vi "Main.vi"() -> ()   [LabVIEW 2017]
uses:
  State/state_R.ctl
  <vilib>/daq.io/daq.io LabVIEW API/_typedefs/daqio-Credentials.ctl
  <vilib>/myRIO/Instrument Drivers/Onboard IO/DIO/typedefs/DIO Reference.ctl
  <vilib>/myRIO/Common/Instrument Driver Framework/Utilities/typedefs/myRIO Generic Hardware Reference.ctl
  <vilib>/myRIO/Common/Instrument Driver Framework/Utilities/typedefs/Hardware Version Enum.ctl
  <vilib>/myRIO/Common/Instrument Driver Framework/Utilities/typedefs/myRIO v1.0 Reference.ctl
  <vilib>/myRIO/Common/Instrument Driver Framework/Utilities/typedefs/Generic FPGA Reference.ctl
  <vilib>/myRIO/Common/Instrument Driver Framework/myRIO v1.0/DIO/typedefs/DIO Channels List.ctl
  <vilib>/myRIO/Common/Instrument Driver Framework/myRIO v1.0/DIO/typedefs/DIO Channels Enum.ctl
  <vilib>/userdefined/High Color/nirio_resource_hc.ctl
  <vilib>/myRIO/Common/Instrument Driver Framework/myRIO v1.0/DIO/vis/myRIO v1.1 Open DIO.vi
  <vilib>/myRIO/Common/Instrument Driver Framework/Utilities/vis/Validate Channels.vi
  <vilib>/myRIO/Common/Instrument Driver Framework/myRIO v1.0/DIO/vis/myRIO v1.0 Reserve DIO.vi
  <vilib>/myRIO/Common/Instrument Driver Framework/myRIO v1.0/DIO/vis/myRIO v1.0 Close DIO.vi
  <vilib>/myRIO/Common/Instrument Driver Framework/myRIO v1.0/Resource Manager/vis/myRIO v1.0 Reserve Channel List.vi
  <vilib>/myRIO/Common/Instrument Driver Framework/myRIO v1.0/DIO/vis/myRIO v1.0 Build MUX Configuration DIO.vi
  <vilib>/myRIO/Common/Instrument Driver Framework/myRIO v1.0/DIO/vis/myRIO v1.0 Unreserve DIO.vi
  <vilib>/myRIO/Common/Instrument Driver Framework/myRIO v1.0/Resource Manager/vis/myRIO v1.0 Reserve Channel.vi
  <vilib>/myRIO/Common/Instrument Driver Framework/myRIO v1.0/Resource Manager/vis/myRIO v1.0 Unreserve Channel.vi
  <vilib>/myRIO/Common/Instrument Driver Framework/myRIO v1.0/Resource Manager/vis/myRIO v1.0 Create Configuration List.vi
  <vilib>/myRIO/Common/Instrument Driver Framework/myRIO v1.0/Resource Manager/vis/myRIO v1.0 Unreserve Channel List.vi
  <vilib>/myRIO/Common/Instrument Driver Framework/myRIO v1.0/Resource Manager/vis/myRIO v1.0 Build Mutex Name.vi
  <vilib>/Utility/VariantDataType/GetNumericInfo.vi
  <vilib>/Utility/error.llb/Error Cluster From Error Code.vi
  <vilib>/myRIO/Common/Instrument Driver Framework/myRIO v1.0/myRIO v1.1 Open.vi
  <vilib>/myRIO/Common/Instrument Driver Framework/Utilities/vis/IO Manager.vi
  <vilib>/myRIO/Common/Instrument Driver Framework/Utilities/vis/Configuration Manager.vi
  <vilib>/myRIO/Common/Instrument Driver Framework/myRIO v1.0/Resource Manager/vis/myRIO v1.0 Configure IO.vi
  <vilib>/myRIO/Common/Instrument Driver Framework/myRIO v1.0/myRIO v1.0 Close.vi
  Function/Global_pH.vi
  <vilib>/daq.io/daq.io LabVIEW API/_subs/daqio_Write_Single.vi
  <vilib>/myRIO/Common/Instrument Driver Framework/myRIO v1.0/DIO/vis/myRIO v1.0 Read DIO.vi
  <vilib>/myRIO/Common/Instrument Driver Framework/myRIO v1.0/DIO/vis/myRIO v1.0 Shutdown DIO.vi
  <vilib>/myRIO/Common/Instrument Driver Framework/myRIO v1.0/DIO/vis/myRIO v1.0 Write DIO.vi
  <vilib>/myRIO/Instrument Drivers/Onboard IO/DIO/vis/myRIO DIO Open.xnode
  <vilib>/myRIO/Instrument Drivers/Onboard IO/DIO/DIO.lvlib
  <vilib>/daq.io/daq.io LabVIEW API/daqio minimal.lvlib
panel:
  in  "分割面板":enum32{"控制面板"}(tab)
  out "pH 感測器狀態異常燈號":bool
  out "pH 感測器壽命":dbl
  out "溫度(°C)":dbl
  out "溫度過高":bool
  out "溫度過低":bool
  out "溶氧飽和度過高":bool
  out "溶氧飽和度過低":bool
  in  "TEM 上限":dbl
  in  "TEM 下限":dbl
  in  "DO 上限(%)":dbl
  in  "DO 下限(%)":dbl
  out "Work":bool
  out "FREE":bool
  out "Dangerous_Work":bool
  in  "登陸設定":T1
  out "過酸":bool
  out "過鹼":bool
  in  "pH 下限":dbl
  in  "pH 上限":dbl
  out "小時":i32
  out "分":i32
  in  "量測時間設定(min)_3":i32
  in  "量測時間設定(24hr)_3":i32
  in  "量測時間設定(min)_2":i32
  in  "量測時間設定(24hr)_2":i32
  in  "量測時間設定(min)_1":i32
  in  "量測時間設定(24hr)_1":i32
  in  "控制模式":enum16{"自動", "手動"}(ring)
  in  "狀態暫停":bool
  out "LS5":bool
  out "LS4":bool
  out "LS3":bool
  out "LS2":bool
  out "LS1":bool
  in  "開始":bool
  in  "晾乾 秒數設定 (s)":dbl
  out "目前狀態":T2
  in  "pH 秒數設定(s)":dbl
  in  "噴水 秒數設定 (s)":dbl
  in  "程式終止":bool
  in  "停止動作":bool
  in  "水平-伸":bool
  in  "水平-縮":bool
  in  "垂直-降":bool
  in  "垂直-升":bool
  out "pH值":dbl
  out "量測計數(s)":dbl
  out "噴水計數(s)":dbl
  out "晾乾計數":dbl
  out "DO值(%)":dbl
  # "Automatic measurement system based on IoT"
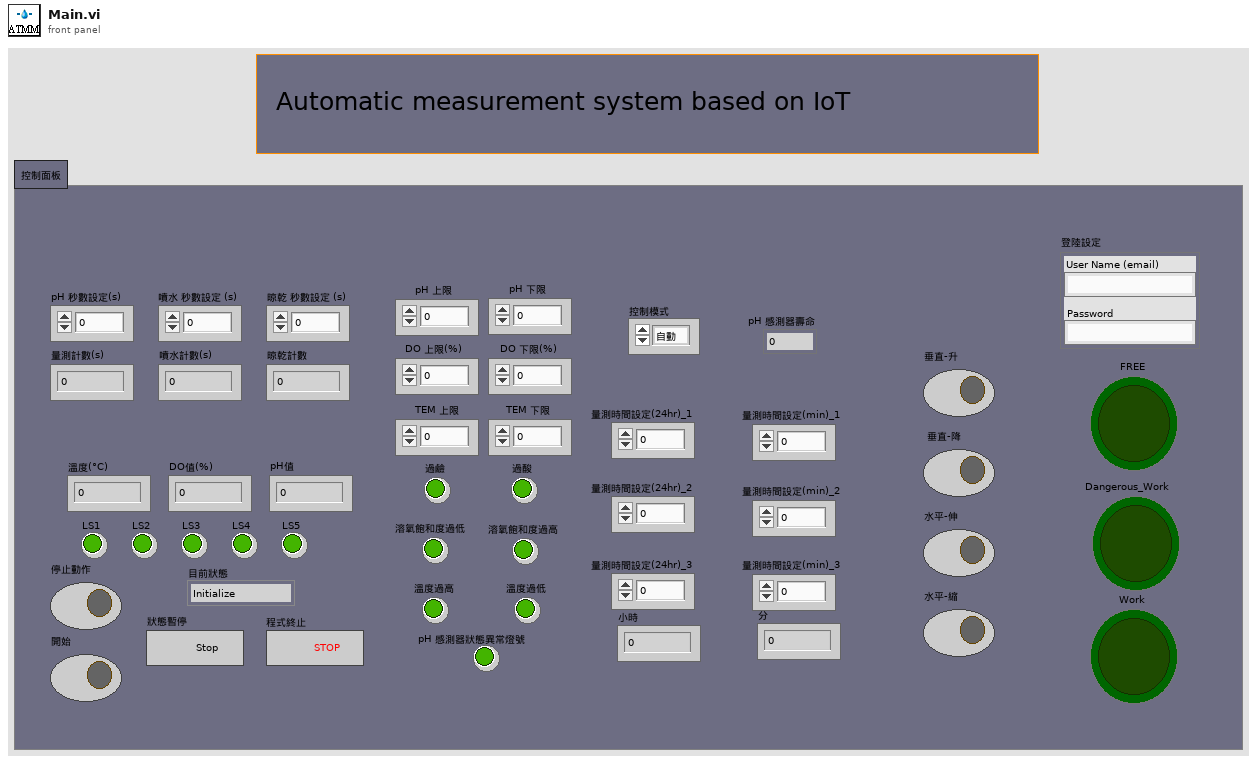
[diagram p1: front panel]
types:
  T1 = typedef "daqio minimal.lvlib/daqio-Credentials.ctl" = cluster{"User Name (email)":string, "Password":string}
  T2 = typedef "state_R.ctl" = enum16{"Initialize", "State 1", "State 2", "State 3", "State 4", "State 5", "State 6", "State 7", "State 8", "State 9", "UP", "DOWN", "EXTEND", "BACK", "Reset", "Process", "PAUSE", "Report", "Halt", "Shutdown"}
  T3 = typedef "daqio minimal.lvlib/daqio-Type.ctl" = cluster{"daq.io ref":T4, "daq.io API Base":string, "Device Key":string, "Account ID":string, "online":bool, "SSL":bool, "buffer":bool}
  T4 = typedef "LabVIEWHTTPClient.lvlib/ClientHandle.ctl" = refnum<k1>
  T5 = typedef "DIO.lvlib/DIO Reference.ctl" = cluster{"myRIO Reference":T6, "DIO Channels List":T10}
  T6 = typedef "myRIO Generic Hardware Reference.ctl" = cluster{"myRIO Model":T7, "myRIO Hardware Reference":T8}
  T7 = typedef "Hardware Version Enum.ctl" = enum16{"Unknown", "myRIO-1900", "myRIO-1950", "roboRIO", "NI ELVIS RIO CM"}
  T8 = typedef "myRIO v1.0 Reference.ctl" = cluster{"Generic FPGA Reference":T9, "Allow multiple opens":bool}
  T9 = typedef "Generic FPGA Reference.ctl" = refnum<k20>
  T10 = typedef "DIO Channels List.ctl" = T11[]
  T11 = typedef "DIO Channels Enum.ctl" = enum16{"Not Connected", "C/DIO0", "C/DIO1", "C/DIO2", "C/DIO3", "C/DIO4", "C/DIO5", "C/DIO6", "C/DIO7", "A/DIO0", "A/DIO1", "A/DIO2", "A/DIO3", "A/DIO4", "A/DIO5", "A/DIO6", "A/DIO7", "A/DIO8", "A/DIO9", "A/DIO10", "A/DIO11", "A/DIO12", "A/DIO13", "A/DIO14", "A/DIO15", "B/DIO0", "B/DIO1", "B/DIO2", "B/DIO3", "B/DIO4", "B/DIO5", "B/DIO6", "B/DIO7", "B/DIO8", "B/DIO9", "B/DIO10", "B/DIO11", "B/DIO12", "B/DIO13", "B/DIO14", "B/DIO15", "LED0", "LED1", "LED2", "LED3", "Button0", "DIO/DIO0", "DIO/DIO1", "DIO/DIO2", "DIO/DIO3", "DIO/DIO4", "DIO/DIO5", "DIO/DIO6", "DIO/DIO7", "DIO/DIO8", "DIO/DIO9", "SPI/CS0", "SPI/CS1", "SPI/CS2", "SPI/CS3", "LED RADIO (Green)", "LED RADIO (Red)", "LED COMM (Green)", "LED COMM (Red)", "LED MODE (Green)", "LED MODE (Red)"}
  T12 = typedef "LVDateTimeRec.ctl" = cluster{"fractional second":dbl, "second":i32, "minute":i32, "hour":i32, "day of month":i32, "month":i32, "year":i32, "day of week":i32, "day of year":i32, "DST":i32}
  T13 = typedef "state_D.ctl" = enum16{"Halt", "Start", "LS1", "LS2", "LS3", "LS4", "LS5", "UP", "DOWN", "EXTEND", "BACK", "Stop", "Pause"}
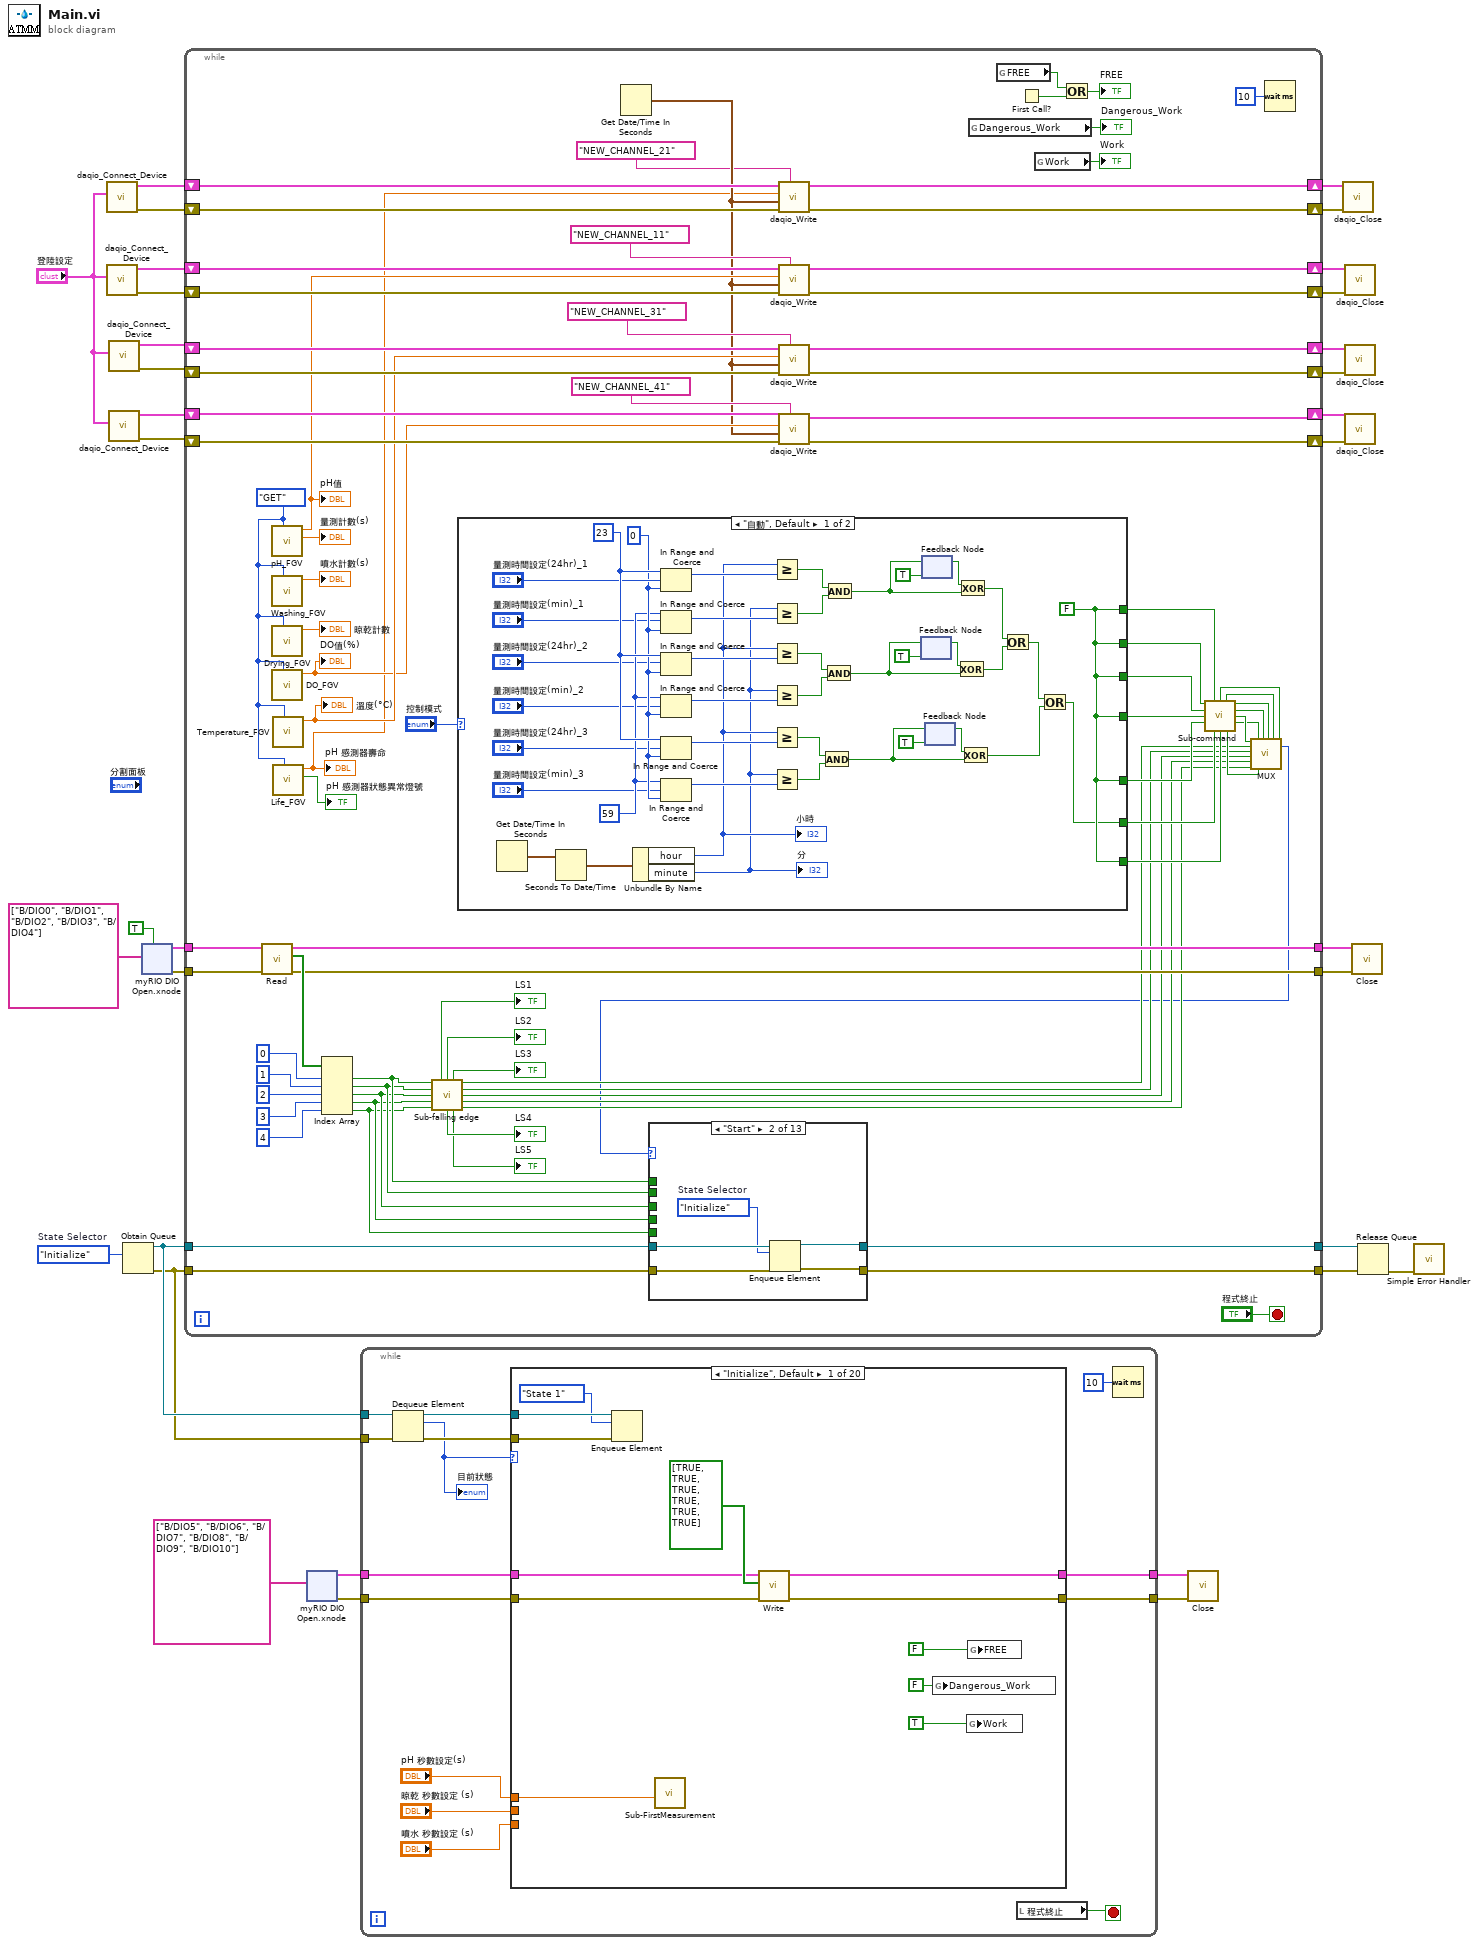
[diagram p0: block diagram]
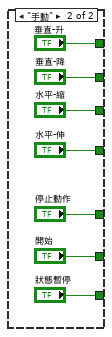
[diagram p2: hidden frame]
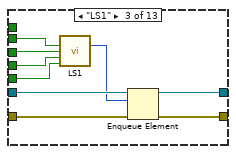
[diagram p4: hidden frame]
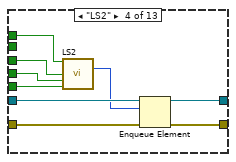
[diagram p5: hidden frame]
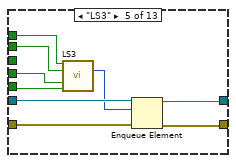
[diagram p6: hidden frame]
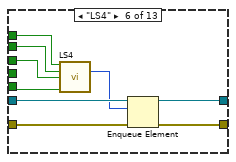
[diagram p7: hidden frame]
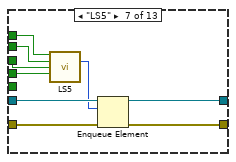
[diagram p8: hidden frame]
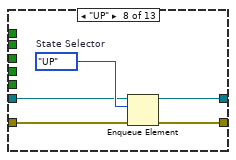
[diagram p9: hidden frame]
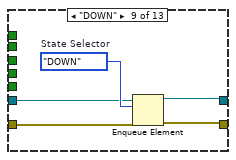
[diagram p10: hidden frame]
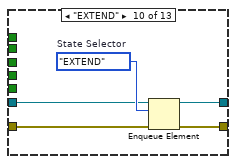
[diagram p11: hidden frame]
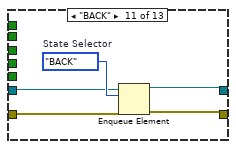
[diagram p12: hidden frame]
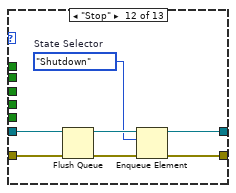
[diagram p13: hidden frame]
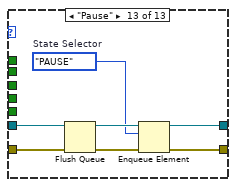
[diagram p14: hidden frame]
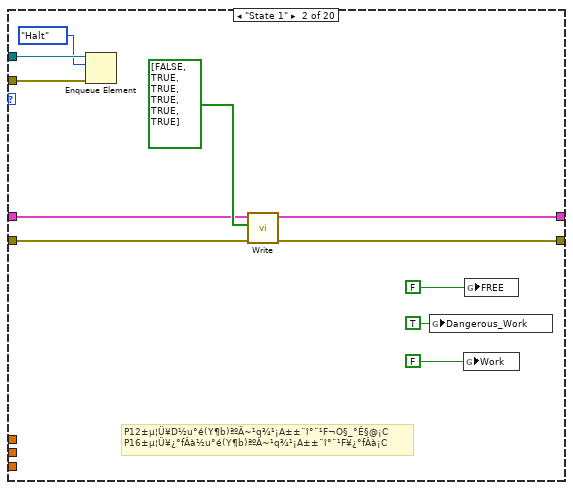
[diagram p15: hidden frame]
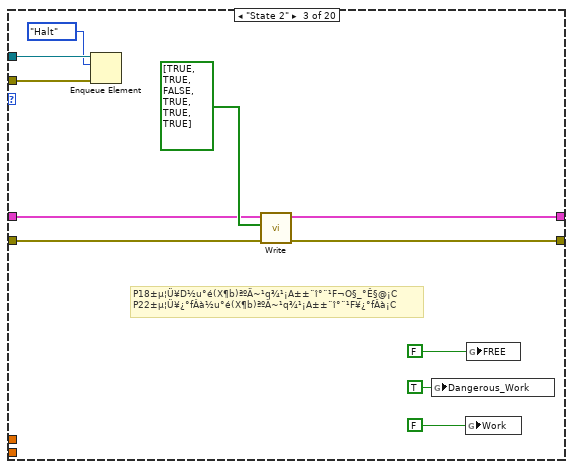
[diagram p16: hidden frame]
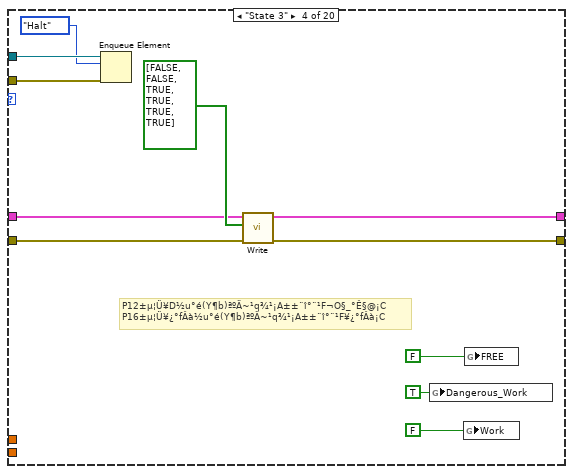
[diagram p17: hidden frame]
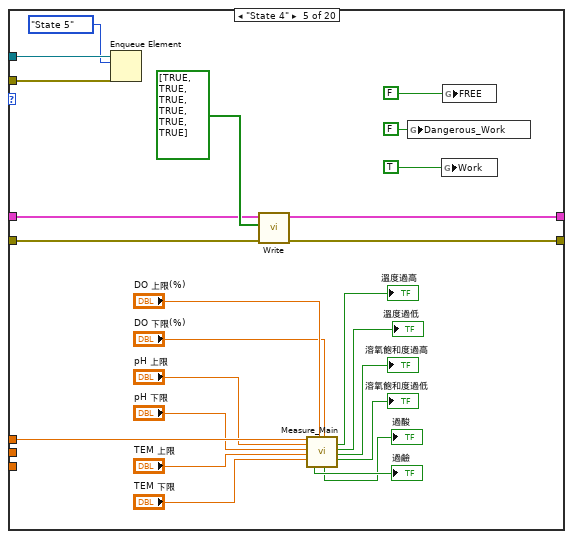
[diagram p18: hidden frame]
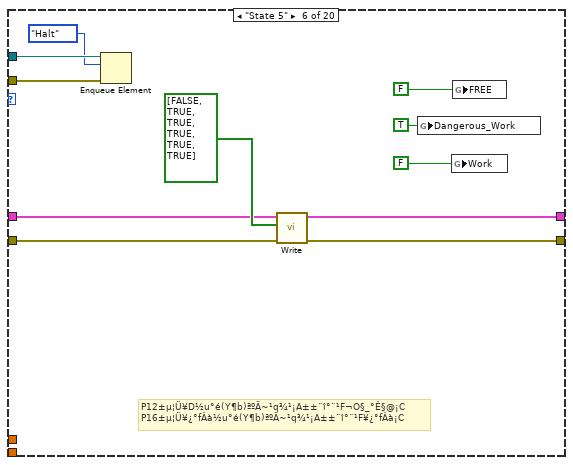
[diagram p19: hidden frame]
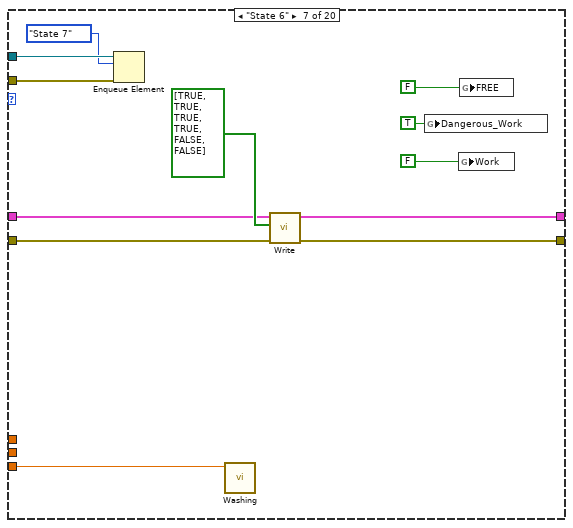
[diagram p20: hidden frame]
diagram:
  w34 = state_R."Initialize"  # State Selector
  n1 = call <vilib>:"daqio_Connect_Device.vi"("Credentials"="登陸設定") -> ("error out"=w4:errorcluster, "daq.io type out"=w5:T3)  [unwired: 8 in, 1 out]
  n2 = call <vilib>:"daqio_Connect_Device.vi"("Credentials"="登陸設定") -> ("error out"=w16:errorcluster, "daq.io type out"=w17:T3)  [unwired: 8 in, 1 out]
  n3 = call <vilib>:"daqio_Connect_Device.vi"("Credentials"="登陸設定") -> ("error out"=w15:errorcluster, "daq.io type out"=w14:T3)  [unwired: 8 in, 1 out]
  n4 = call <vilib>:"daqio_Connect_Device.vi"("Credentials"="登陸設定") -> ("error out"=w12:errorcluster, "daq.io type out"=w13:T3)  [unwired: 8 in, 1 out]
  n5 = Obtain Queue(element data type=w34) -> (queue out=w33:refnum<queue>, error out=w32:errorcluster)  [unwired: 4 in, 1 out]
  n6 = xnode "myRIO DIO Open.xnode"("Allow multiple opens?"=TRUE, "Channel Names"=tag[] ["B/DIO0", "B/DIO1", "B/DIO2", "B/DIO3", "B/DIO4"]) -> ("error out"=w25:errorcluster, "DIO Ref Out"=w26:T5)  [unwired: 1 in]
  n7 = while {
    tunnel: w33 -> [w114]
    tunnel: w32 -> [w113]
    tunnel: [w112] -> w31
    tunnel: [w111] -> w30
    tunnel: w26 -> [w89]
    tunnel: w25 -> [w88]
    tunnel: [w87] -> w24
    tunnel: [w86] -> w23
    shift-right: [w48] -> w11
    shift-left: w17 -> [w51]
    shift-right: [w47] -> w10
    shift-left: w16 -> [w49]
    shift-right: [w52] -> w8
    shift-left: w15 -> [w54]
    shift-right: [w53] -> w9
    shift-left: w14 -> [w55]
    shift-right: [w57] -> w7
    shift-left: w13 -> [w58]
    shift-right: [w56] -> w6
    shift-left: w12 -> [w59]
    shift-right: [w39] -> w3
    shift-left: w5 -> [w41]
    shift-right: [w38] -> w2
    shift-left: w4 -> [w40]
    stop <- "程式終止" stop-if-true
    w43 = enum16{"SET", "GET"}."GET" ("Command")
    n8 = call <vilib>:"Read.vi"("error in (no error)"=w88, "DIO Ref In"=w89) -> ("error out"=w86:errorcluster, "Values"=w95:bool[], "DIO Ref Out"=w87:T5)  [unwired: 7 in]
    n9 = call "pH_FGV.vi"("Command"=w43) -> ("Elapsed_Time(s)_OUT"=→"量測計數(s)":dbl, "pH_Value_OUT"=w46:dbl)  [unwired: 8 in, 1 out]
    "pH值" <- w46
    n10 = call "Washing_FGV.vi"("Command"=w43) -> ("Elased_Time(s)_OUT"=→"噴水計數(s)":dbl)  [unwired: 9 in, 1 out]
    n11 = call "Drying_FGV.vi"("Command"=w43) -> ("Elapsed_Time(s)_OUT"=→"晾乾計數":dbl)  [unwired: 9 in, 1 out]
    n12 = call "DO_FGV.vi"("Command"=w43) -> ("DO_Value_OUT"=w44:dbl)  [unwired: 9 in, 1 out]
    "DO值(%)" <- w44
    n13 = call "Temperature_FGV.vi"("Command"=w43) -> ("Temperature_OUT"=w45:dbl)  [unwired: 9 in, 1 out]
    "溫度(°C)" <- w45
    n14 = call "Life_FGV.vi"("Command"=w43) -> ("Error_OUT"=→"pH 感測器狀態異常燈號":bool, "Life_Value_OUT"=w35:dbl)  [unwired: 8 in, 1 out]
    "pH 感測器壽命" <- w35
    n15 = Index Array(array=w95, index #1=0 ("index"), index #2=1 ("index"), index #3=2 ("index"), index #4=3 ("index"), index #5=4 ("index")) -> (element #1=w71:bool, element #2=w70:bool, element #3=w69:bool, element #4=w68:bool, element #5=w67:bool)
    n16 = call "Sub-falling edge.vi"("LS1_DI"=w71, "LS2_DI"=w70, "LS3_DI"=w69, "LS4_DI"=w68, "LS5_DI"=w67) -> ("LS1_Shift"=→"LS1":bool, "LS2_Shift"=→"LS2":bool, "LS3_Shift"=→"LS3":bool, "LS1_DO"=w80:bool, "LS2_DO"=w79:bool, "LS3_DO"=w78:bool, "LS4_DO"=w77:bool, "LS4_Shift"=→"LS4":bool, "LS5_Shift"=→"LS5":bool, "LS5_DO"=w76:bool)  [unwired: 1 in]
    n17 = case shown="\"自動\", Default" "控制模式" {
      tunnel: [w120 "開始"] -> w110
      tunnel: [w156 "狀態暫停"] -> w109
      tunnel: [w156 "停止動作"] -> w107
      tunnel: [w156 "水平-伸"] -> w105
      tunnel: [w156 "水平-縮"] -> w104
      tunnel: [w156 "垂直-降"] -> w103
      tunnel: [w156 "垂直-升"] -> w102
      frame "自動", Default {
        w150 = 59
        w151 = 0
        w153 = 23
        w156 = FALSE ("垂直-升")
        n18 = Get Date/Time In Seconds() -> (seconds since 1Jan1904=w155:timestamp)
        n19 = Seconds To Date/Time(time stamp (now)=w155) -> (date time rec=w154:T12)  [unwired: 1 in]
        n20 = Unbundle By Name(w154) -> ("hour"=w138:i32, "minute"=w137:i32)
        "小時" <- w138
        "分" <- w137
        n21 = In Range and Coerce(upper limit=w153, x="量測時間設定(24hr)_1", lower limit=w151) -> (coerced(x)=w144:i32)  [unwired: 1 out]
        n22 = In Range and Coerce(upper limit=w150, x="量測時間設定(min)_1", lower limit=w151) -> (coerced(x)=w141:i32)  [unwired: 1 out]
        n23 = In Range and Coerce(upper limit=w153, x="量測時間設定(24hr)_2", lower limit=w151) -> (coerced(x)=w143:i32)  [unwired: 1 out]
        n24 = In Range and Coerce(upper limit=w150, x="量測時間設定(min)_2", lower limit=w151) -> (coerced(x)=w140:i32)  [unwired: 1 out]
        n25 = In Range and Coerce(upper limit=w153, x="量測時間設定(24hr)_3", lower limit=w151) -> (coerced(x)=w142:i32)  [unwired: 1 out]
        n26 = In Range and Coerce(upper limit=w150, x="量測時間設定(min)_3", lower limit=w151) -> (coerced(x)=w139:i32)  [unwired: 1 out]
        n27 = Greater Or Equal?(x=w138, y=w144) -> (x >= y?=w136:bool)
        n28 = Greater Or Equal?(x=w137, y=w141) -> (x >= y?=w135:bool)
        n29 = Greater Or Equal?(x=w138, y=w143) -> (x >= y?=w134:bool)
        n30 = Greater Or Equal?(x=w137, y=w140) -> (x >= y?=w133:bool)
        n31 = Greater Or Equal?(x=w138, y=w142) -> (x >= y?=w132:bool)
        n32 = Greater Or Equal?(x=w137, y=w139) -> (x >= y?=w131:bool)
        n33 = And(x=w132, y=w131) -> (x .and. y?=w117:bool)
        n34 = And(x=w134, y=w133) -> (x .and. y?=w118:bool)
        n35 = And(x=w136, y=w135) -> (x .and. y?=w119:bool)
        n36 = feedback #1(TRUE ("DI Value")) -> (w127:bool)
        n37 = feedback-in #1(w118) -> ()
        n38 = feedback #2(TRUE ("DI Value")) -> (w130:bool)
        n39 = feedback-in #2(w119) -> ()
        n40 = feedback #3(TRUE ("DI Value")) -> (w125:bool)
        n41 = feedback-in #3(w117) -> ()
        n42 = Exclusive Or(1:w118, 2:w127) -> (0:w123:bool)
        n43 = Exclusive Or(1:w119, 2:w130) -> (0:w128:bool)
        n44 = Exclusive Or(1:w117, 2:w125) -> (0:w121:bool)
        n45 = Or(x=w128, y=w123) -> (x .or. y?=w122:bool)
        n46 = Or(x=w122, y=w121) -> (x .or. y?=w120:bool)
      }
      frame "手動" {
      }
    }
    n47 = Get Date/Time In Seconds() -> (seconds since 1Jan1904=w37:timestamp)
    n48 = call-poly <vilib>:"daqio_Write.vi"("daq.io Device Channel Key"="NEW_CHANNEL_21", "error in (no error)"=w40, "timestamp"=w37, "value"=w35, "daq.io type in"=w41) -> ("error out"=w38:errorcluster, "daq.io type out"=w39:T3)  [unwired: 5 in]
    n49 = call-poly <vilib>:"daqio_Write.vi"("daq.io Device Channel Key"="NEW_CHANNEL_11", "error in (no error)"=w49, "timestamp"=w37, "value"=w46, "daq.io type in"=w51) -> ("error out"=w47:errorcluster, "daq.io type out"=w48:T3)  [unwired: 5 in]
    n50 = call-poly <vilib>:"daqio_Write.vi"("daq.io Device Channel Key"="NEW_CHANNEL_31", "error in (no error)"=w54, "timestamp"=w37, "value"=w45, "daq.io type in"=w55) -> ("error out"=w52:errorcluster, "daq.io type out"=w53:T3)  [unwired: 5 in]
    n51 = call-poly <vilib>:"daqio_Write.vi"("daq.io Device Channel Key"="NEW_CHANNEL_41", "error in (no error)"=w59, "timestamp"=w37, "value"=w44, "daq.io type in"=w58) -> ("error out"=w56:errorcluster, "daq.io type out"=w57:T3)  [unwired: 5 in]
    n52 = global read "Global_pH.vi" "Dangerous_Work"() -> (→"Dangerous_Work":bool)
    n53 = global read "Global_pH.vi" "FREE"() -> (w64:bool)
    n54 = First Call?() -> (First Call?: T/F=w66:bool)
    n55 = global read "Global_pH.vi" "Work"() -> (→"Work":bool)
    n56 = Or(x=w64, y=w66) -> (x .or. y?=→"FREE":bool)
    n57 = call "Sub-command.vi"("垂直-降"=w103, "垂直-升"=w102, "水平-縮"=w104, "水平-伸"=w105, "停止動作"=w107, "開始"=w110, "暫停"=w109) -> ("水平-縮_輸出"=w99:bool, "水平-伸_輸出"=w100:bool, "垂直-降_輸出"=w101:bool, "垂直-升_輸出"=w98:bool, "開始_輸出"=w116:bool, "停止動作_輸出"=w106:bool, "暫停_輸出"=w115:bool)  [unwired: 2 in]
    n58 = call "MUX.vi"("Start"=w116, "LS1"=w80, "LS2"=w79, "LS3"=w78, "LS4"=w77, "LS5"=w76, "Pause"=w106, "Stop"=w115, "UP"=w98, "DOWN"=w101, "EXTEND"=w100, "BACK"=w99) -> ("Enum"=w75:T13)  [unwired: 7 in]
    n59 = case shown="\"Start\"" w75 {
      tunnel: w114 -> [w165 w170 w179 w188 w197 w206 w215 w219 w224 w229 w234 w242 w246]
      tunnel: w113 -> [w164 w169 w178 w187 w196 w205 w213 w218 w223 w228 w233 w241 w245]
      tunnel: [w165 w167 w176 w185 w194 w203 w212 w217 w222 w227 w232 w238 w244] -> w112
      tunnel: [w164 w166 w175 w184 w193 w202 w211 w216 w221 w226 w231 w237 w243] -> w111
      tunnel: w71 -> [_ _ _ w183 w192 w201 w210 _ _ _ _ _ _]
      tunnel: w70 -> [_ _ w174 _ w191 w200 w209 _ _ _ _ _ _]
      tunnel: w69 -> [_ _ w173 w182 _ w199 w208 _ _ _ _ _ _]
      tunnel: w68 -> [_ _ w172 w181 w190 _ w207 _ _ _ _ _ _]
      tunnel: w67 -> [_ _ w171 w180 w189 w198 _ _ _ _ _ _ _]
      frame "Halt", Default {
      }
      frame "Start" {
        w168 = state_R."Initialize"  # State Selector
        n60 = Enqueue Element(queue=w170, element=w168, error in (no error)=w169) -> (queue out=w167:refnum<queue>, error out=w166:errorcluster)  [unwired: 1 in, 1 out]
      }
      frame "LS1" {
        n61 = call "LS1.vi"("LS2"=w174, "LS3"=w173, "LS4"=w172, "LS5"=w171) -> ("State Selector"=w177:T2)  [unwired: 11 in]
        n62 = Enqueue Element(queue=w179, element=w177, error in (no error)=w178) -> (queue out=w176:refnum<queue>, error out=w175:errorcluster)  [unwired: 1 in, 1 out]
      }
      frame "LS2" {
        n63 = call "LS2.vi"("LS1"=w183, "LS3"=w182, "LS4"=w181, "LS5"=w180) -> ("State Selector"=w186:T2)  [unwired: 11 in]
        n64 = Enqueue Element(queue=w188, element=w186, error in (no error)=w187) -> (queue out=w185:refnum<queue>, error out=w184:errorcluster)  [unwired: 1 in, 1 out]
      }
      frame "LS3" {
        n65 = call "LS3.vi"("LS1"=w192, "LS2"=w191, "LS4"=w190, "LS5"=w189) -> ("State Selector"=w195:T2)  [unwired: 11 in]
        n66 = Enqueue Element(queue=w197, element=w195, error in (no error)=w196) -> (queue out=w194:refnum<queue>, error out=w193:errorcluster)  [unwired: 1 in, 1 out]
      }
      frame "LS4" {
        n67 = call "LS4.vi"("LS1"=w201, "LS2"=w200, "LS3"=w199, "LS5"=w198) -> ("State Selector"=w204:T2)  [unwired: 11 in]
        n68 = Enqueue Element(queue=w206, element=w204, error in (no error)=w205) -> (queue out=w203:refnum<queue>, error out=w202:errorcluster)  [unwired: 1 in, 1 out]
      }
      frame "LS5" {
        n69 = call "LS5.vi"("LS1"=w210, "LS2"=w209, "LS3"=w208, "LS4"=w207) -> ("State Selector"=w214:T2)  [unwired: 11 in]
        n70 = Enqueue Element(queue=w215, element=w214, error in (no error)=w213) -> (queue out=w212:refnum<queue>, error out=w211:errorcluster)  [unwired: 1 in, 1 out]
      }
      frame "UP" {
        w220 = state_R."UP"  # State Selector
        n71 = Enqueue Element(queue=w219, element=w220, error in (no error)=w218) -> (queue out=w217:refnum<queue>, error out=w216:errorcluster)  [unwired: 1 in, 1 out]
      }
      frame "DOWN" {
        w225 = state_R."DOWN"  # State Selector
        n72 = Enqueue Element(queue=w224, element=w225, error in (no error)=w223) -> (queue out=w222:refnum<queue>, error out=w221:errorcluster)  [unwired: 1 in, 1 out]
      }
      frame "EXTEND" {
        w230 = state_R."EXTEND"  # State Selector
        n73 = Enqueue Element(queue=w229, element=w230, error in (no error)=w228) -> (queue out=w227:refnum<queue>, error out=w226:errorcluster)  [unwired: 1 in, 1 out]
      }
      frame "BACK" {
        w235 = state_R."BACK"  # State Selector
        n74 = Enqueue Element(queue=w234, element=w235, error in (no error)=w233) -> (queue out=w232:refnum<queue>, error out=w231:errorcluster)  [unwired: 1 in, 1 out]
      }
      frame "Stop" {
        w236 = state_R."Shutdown"  # State Selector
        n75 = Flush Queue(queue=w242, error in (no error)=w241) -> (queue out=w240:refnum<queue>, error out=w239:errorcluster)  [unwired: 1 out]
        n76 = Enqueue Element(queue=w240, element=w236, error in (no error)=w239) -> (queue out=w238:refnum<queue>, error out=w237:errorcluster)  [unwired: 1 in, 1 out]
      }
      frame "Pause" {
        w247 = state_R."PAUSE"  # State Selector
        n77 = Flush Queue(queue=w246, error in (no error)=w245) -> (queue out=w249:refnum<queue>, error out=w248:errorcluster)  [unwired: 1 out]
        n78 = Enqueue Element(queue=w249, element=w247, error in (no error)=w248) -> (queue out=w244:refnum<queue>, error out=w243:errorcluster)  [unwired: 1 in, 1 out]
      }
    }
    n79 = Wait (ms)(milliseconds to wait=u32 10) -> ()  [unwired: 1 out]
  }
  n80 = xnode "myRIO DIO Open.xnode"("Channel Names"=tag[] ["B/DIO5", "B/DIO6", "B/DIO7", "B/DIO8", "B/DIO9", "B/DIO10"]) -> ("error out"=w21:errorcluster, "DIO Ref Out"=w22:T5)  [unwired: 2 in]
  n81 = while {
    tunnel: w33 -> [w259]
    tunnel: w32 -> [w258]
    tunnel: w22 -> [w256]
    tunnel: w21 -> [w255]
    tunnel: [w254] -> w20
    tunnel: [w253] -> w19
    stop <- w257 stop-if-true
    n82 = Dequeue Element(queue=w259, error in (no error)=w258) -> (queue out=w263:refnum<queue>, element=w261:T2, error out=w262:errorcluster)  [unwired: 1 in, 1 out]
    "目前狀態" <- w261
    n83 = case shown="\"Initialize\", Default" w261 {
      tunnel: w263 -> [w275 w286 w297 w308 w332 w343 w355 w367 w378 w389 w399 w410 w421 w432 w441 w446 w453 w462 _ _]
      tunnel: w262 -> [w274 w285 w296 w307 w331 w342 w354 w366 w377 w388 w398 w409 w420 w431 w440 w445 w452 w461 _ _]
      tunnel: "pH 秒數設定(s)" -> [w272 _ _ _ w329 _ _ _ _ _ _ _ _ _ _ _ _ _ _ _]
      tunnel: "晾乾 秒數設定 (s)" -> [_ _ _ _ _ _ _ w364 _ _ _ _ _ _ _ _ _ _ _ _]
      tunnel: "噴水 秒數設定 (s)" -> [_ _ _ _ _ _ w352 _ _ _ _ _ _ _ _ _ _ _ _ _]
      tunnel: w256 -> [w270 w282 w293 w304 w323 w339 w350 w362 w374 w385 w396 w407 w418 w429 w437 w443 w450 w458 w464 w471]
      tunnel: w255 -> [w269 w281 w292 w303 w322 w338 w349 w361 w373 w384 w395 w406 w417 w428 w436 w442 w449 w457 w463 w470]
      tunnel: [w268 w280 w291 w302 w321 w337 w348 w360 w372 w383 w394 w405 w416 w427 w435 w443 w448 w456 w464 w469] -> w254
      tunnel: [w267 w279 w290 w301 w320 w336 w347 w359 w371 w382 w393 w404 w415 w426 w434 w442 w447 w455 w463 w468] -> w253
      frame "Initialize", Default {
        n84 = Enqueue Element(queue=w275, element=state_R."State 1" ("State Selector"), error in (no error)=w274) -> ()  [unwired: 1 in, 3 out]
        n85 = call "Sub-FirstMeasurement.vi"("time target (s)"=w272) -> ()  [unwired: 8 in, 3 out]
        n86 = call <vilib>:"Write.vi"("error in (no error)"=w269, "Values"=bool[] [TRUE, TRUE, TRUE, TRUE, TRUE, TRUE], "DIO Ref In"=w270) -> ("error out"=w267:errorcluster, "DIO Ref Out"=w268:T5)  [unwired: 6 in]
        n87 = global write "Global_pH.vi" "Dangerous_Work"(FALSE ("Dangerous_Work")) -> ()
        n88 = global write "Global_pH.vi" "Work"(TRUE ("Dangerous_Work")) -> ()
        n89 = global write "Global_pH.vi" "FREE"(FALSE ("Dangerous_Work")) -> ()
      }
      frame "State 1" {
        # "P12±µ¦Ü¥D½u°é(Y¶b)ªºÄ~¹q¾¹¡A±±¨î°¨¹F¬O§_°Ê§@¡C\nP16±µ¦Ü¥¿°fÂà½u°é(Y¶b)ªºÄ~¹q¾¹¡A±±¨î°¨¹F¥¿°fÂà¡C"
        n90 = Enqueue Element(queue=w286, element=state_R."Halt" ("State Selector"), error in (no error)=w285) -> ()  [unwired: 1 in, 3 out]
        n91 = call <vilib>:"Write.vi"("error in (no error)"=w281, "Values"=bool[] [FALSE, TRUE, TRUE, TRUE, TRUE, TRUE], "DIO Ref In"=w282) -> ("error out"=w279:errorcluster, "DIO Ref Out"=w280:T5)  [unwired: 6 in]
        n92 = global write "Global_pH.vi" "Dangerous_Work"(TRUE ("Dangerous_Work")) -> ()
        n93 = global write "Global_pH.vi" "Work"(FALSE ("Dangerous_Work")) -> ()
        n94 = global write "Global_pH.vi" "FREE"(FALSE ("Dangerous_Work")) -> ()
      }
      frame "State 2" {
        # "P18±µ¦Ü¥D½u°é(X¶b)ªºÄ~¹q¾¹¡A±±¨î°¨¹F¬O§_°Ê§@¡C\nP22±µ¦Ü¥¿°fÂà½u°é(X¶b)ªºÄ~¹q¾¹¡A±±¨î°¨¹F¥¿°fÂà¡C"
        n95 = Enqueue Element(queue=w297, element=state_R."Halt" ("State Selector"), error in (no error)=w296) -> ()  [unwired: 1 in, 3 out]
        n96 = call <vilib>:"Write.vi"("error in (no error)"=w292, "Values"=bool[] [TRUE, TRUE, FALSE, TRUE, TRUE, TRUE], "DIO Ref In"=w293) -> ("error out"=w290:errorcluster, "DIO Ref Out"=w291:T5)  [unwired: 6 in]
        n97 = global write "Global_pH.vi" "Dangerous_Work"(TRUE ("Dangerous_Work")) -> ()
        n98 = global write "Global_pH.vi" "Work"(FALSE ("Dangerous_Work")) -> ()
        n99 = global write "Global_pH.vi" "FREE"(FALSE ("Dangerous_Work")) -> ()
      }
      frame "State 3" {
        # "P12±µ¦Ü¥D½u°é(Y¶b)ªºÄ~¹q¾¹¡A±±¨î°¨¹F¬O§_°Ê§@¡C\nP16±µ¦Ü¥¿°fÂà½u°é(Y¶b)ªºÄ~¹q¾¹¡A±±¨î°¨¹F¥¿°fÂà¡C"
        n100 = Enqueue Element(queue=w308, element=state_R."Halt" ("State Selector"), error in (no error)=w307) -> ()  [unwired: 1 in, 3 out]
        n101 = call <vilib>:"Write.vi"("error in (no error)"=w303, "Values"=bool[] [FALSE, FALSE, TRUE, TRUE, TRUE, TRUE], "DIO Ref In"=w304) -> ("error out"=w301:errorcluster, "DIO Ref Out"=w302:T5)  [unwired: 6 in]
        n102 = global write "Global_pH.vi" "Dangerous_Work"(TRUE ("Dangerous_Work")) -> ()
        n103 = global write "Global_pH.vi" "Work"(FALSE ("Dangerous_Work")) -> ()
        n104 = global write "Global_pH.vi" "FREE"(FALSE ("Dangerous_Work")) -> ()
      }
      frame "State 4" {
        n105 = Enqueue Element(queue=w332, element=state_R."State 5" ("State Selector"), error in (no error)=w331) -> ()  [unwired: 1 in, 3 out]
        n106 = call <vilib>:"Write.vi"("error in (no error)"=w322, "Values"=bool[] [TRUE, TRUE, TRUE, TRUE, TRUE, TRUE], "DIO Ref In"=w323) -> ("error out"=w320:errorcluster, "DIO Ref Out"=w321:T5)  [unwired: 6 in]
        n107 = call "Measure_Main.vi"("time target (s)"=w329, "Upper limit of pH Value"="pH 上限", "Lower limit of pH Value"="pH 下限", "Upper limit of TEM"="TEM 上限", "Lower limit of TEM"="TEM 下限", "Upper limit of DO"="DO 上限(%)", "Lower limit of DO"="DO 下限(%)") -> ("Maximum Alarm_pH"=→"過鹼":bool, "Minumum Alarm_pH"=→"過酸":bool, "Maximum Alarm_TEM"=→"溫度過高":bool, "Minumum Alarm_TEM"=→"溫度過低":bool, "Maximum Alarm_DO"=→"溶氧飽和度過高":bool, "Minumum Alarm_DO"=→"溶氧飽和度過低":bool)  [unwired: 6 in, 1 out]
        n108 = global write "Global_pH.vi" "Dangerous_Work"(FALSE ("Dangerous_Work")) -> ()
        n109 = global write "Global_pH.vi" "Work"(TRUE ("Dangerous_Work")) -> ()
        n110 = global write "Global_pH.vi" "FREE"(FALSE ("Dangerous_Work")) -> ()
      }
      frame "State 5" {
        # "P12±µ¦Ü¥D½u°é(Y¶b)ªºÄ~¹q¾¹¡A±±¨î°¨¹F¬O§_°Ê§@¡C\nP16±µ¦Ü¥¿°fÂà½u°é(Y¶b)ªºÄ~¹q¾¹¡A±±¨î°¨¹F¥¿°fÂà¡C"
        n111 = Enqueue Element(queue=w343, element=state_R."Halt" ("State Selector"), error in (no error)=w342) -> ()  [unwired: 1 in, 3 out]
        n112 = call <vilib>:"Write.vi"("error in (no error)"=w338, "Values"=bool[] [FALSE, TRUE, TRUE, TRUE, TRUE, TRUE], "DIO Ref In"=w339) -> ("error out"=w336:errorcluster, "DIO Ref Out"=w337:T5)  [unwired: 6 in]
        n113 = global write "Global_pH.vi" "Dangerous_Work"(TRUE ("Dangerous_Work")) -> ()
        n114 = global write "Global_pH.vi" "Work"(FALSE ("Dangerous_Work")) -> ()
        n115 = global write "Global_pH.vi" "FREE"(FALSE ("Dangerous_Work")) -> ()
      }
      frame "State 6" {
        n116 = Enqueue Element(queue=w355, element=state_R."State 7" ("State Selector"), error in (no error)=w354) -> ()  [unwired: 1 in, 3 out]
        n117 = call "Washing.vi"("time target (s)"=w352) -> ()  [unwired: 10 in, 1 out]
        n118 = call <vilib>:"Write.vi"("error in (no error)"=w349, "Values"=bool[] [TRUE, TRUE, TRUE, TRUE, FALSE, FALSE], "DIO Ref In"=w350) -> ("error out"=w347:errorcluster, "DIO Ref Out"=w348:T5)  [unwired: 6 in]
        n119 = global write "Global_pH.vi" "Dangerous_Work"(TRUE ("Dangerous_Work")) -> ()
        n120 = global write "Global_pH.vi" "Work"(FALSE ("Dangerous_Work")) -> ()
        n121 = global write "Global_pH.vi" "FREE"(FALSE ("Dangerous_Work")) -> ()
      }
      frame "State 7" {
        n122 = Enqueue Element(queue=w367, element=state_R."State 8" ("State Selector"), error in (no error)=w366) -> ()  [unwired: 1 in, 3 out]
        n123 = call "Drying.vi"("time target (s)"=w364) -> ()  [unwired: 10 in, 1 out]
        n124 = call <vilib>:"Write.vi"("error in (no error)"=w361, "Values"=bool[] [TRUE, TRUE, TRUE, TRUE, TRUE, TRUE], "DIO Ref In"=w362) -> ("error out"=w359:errorcluster, "DIO Ref Out"=w360:T5)  [unwired: 6 in]
        n125 = global write "Global_pH.vi" "Dangerous_Work"(FALSE ("Dangerous_Work")) -> ()
        n126 = global write "Global_pH.vi" "Work"(TRUE ("Dangerous_Work")) -> ()
        n127 = global write "Global_pH.vi" "FREE"(FALSE ("Dangerous_Work")) -> ()
      }
      frame "State 8" {
        # "P18±µ¦Ü¥D½u°é(X¶b)ªºÄ~¹q¾¹¡A±±¨î°¨¹F¬O§_°Ê§@¡C\nP22±µ¦Ü¥¿°fÂà½u°é(X¶b)ªºÄ~¹q¾¹¡A±±¨î°¨¹F¥¿°fÂà¡C"
        n128 = Enqueue Element(queue=w378, element=state_R."Halt" ("State Selector"), error in (no error)=w377) -> ()  [unwired: 1 in, 3 out]
        n129 = call <vilib>:"Write.vi"("error in (no error)"=w373, "Values"=bool[] [TRUE, TRUE, FALSE, FALSE, TRUE, TRUE], "DIO Ref In"=w374) -> ("error out"=w371:errorcluster, "DIO Ref Out"=w372:T5)  [unwired: 6 in]
        n130 = global write "Global_pH.vi" "Dangerous_Work"(TRUE ("Dangerous_Work")) -> ()
        n131 = global write "Global_pH.vi" "Work"(FALSE ("Dangerous_Work")) -> ()
        n132 = global write "Global_pH.vi" "FREE"(FALSE ("Dangerous_Work")) -> ()
      }
      frame "State 9" {
        # "P12±µ¦Ü¥D½u°é(Y¶b)ªºÄ~¹q¾¹¡A±±¨î°¨¹F¬O§_°Ê§@¡C\nP16±µ¦Ü¥¿°fÂà½u°é(Y¶b)ªºÄ~¹q¾¹¡A±±¨î°¨¹F¥¿°fÂà¡C"
        n133 = Enqueue Element(queue=w389, element=state_R."Halt" ("State Selector"), error in (no error)=w388) -> ()  [unwired: 1 in, 3 out]
        n134 = call <vilib>:"Write.vi"("error in (no error)"=w384, "Values"=bool[] [FALSE, FALSE, TRUE, TRUE, TRUE, TRUE], "DIO Ref In"=w385) -> ("error out"=w382:errorcluster, "DIO Ref Out"=w383:T5)  [unwired: 6 in]
        n135 = global write "Global_pH.vi" "Dangerous_Work"(TRUE ("Dangerous_Work")) -> ()
        n136 = global write "Global_pH.vi" "Work"(FALSE ("Dangerous_Work")) -> ()
        n137 = global write "Global_pH.vi" "FREE"(FALSE ("Dangerous_Work")) -> ()
      }
      frame "UP" {
        n138 = Enqueue Element(queue=w399, element=state_R."Halt" ("State Selector"), error in (no error)=w398) -> ()  [unwired: 1 in, 3 out]
        n139 = call <vilib>:"Write.vi"("error in (no error)"=w395, "Values"=bool[] [FALSE, TRUE, TRUE, TRUE, TRUE, TRUE], "DIO Ref In"=w396) -> ("error out"=w393:errorcluster, "DIO Ref Out"=w394:T5)  [unwired: 6 in]
        n140 = global write "Global_pH.vi" "Dangerous_Work"(TRUE ("Dangerous_Work")) -> ()
        n141 = global write "Global_pH.vi" "Work"(FALSE ("Dangerous_Work")) -> ()
        n142 = global write "Global_pH.vi" "FREE"(FALSE ("Dangerous_Work")) -> ()
      }
      frame "DOWN" {
        n143 = Enqueue Element(queue=w410, element=state_R."Halt" ("State Selector"), error in (no error)=w409) -> ()  [unwired: 1 in, 3 out]
        n144 = call <vilib>:"Write.vi"("error in (no error)"=w406, "Values"=bool[] [FALSE, FALSE, TRUE, TRUE, TRUE, TRUE], "DIO Ref In"=w407) -> ("error out"=w404:errorcluster, "DIO Ref Out"=w405:T5)  [unwired: 6 in]
        n145 = global write "Global_pH.vi" "Dangerous_Work"(TRUE ("Dangerous_Work")) -> ()
        n146 = global write "Global_pH.vi" "Work"(FALSE ("Dangerous_Work")) -> ()
        n147 = global write "Global_pH.vi" "FREE"(FALSE ("Dangerous_Work")) -> ()
      }
      frame "EXTEND" {
        n148 = Enqueue Element(queue=w421, element=state_R."Halt" ("State Selector"), error in (no error)=w420) -> ()  [unwired: 1 in, 3 out]
        n149 = call <vilib>:"Write.vi"("error in (no error)"=w417, "Values"=bool[] [TRUE, TRUE, FALSE, FALSE, TRUE, TRUE], "DIO Ref In"=w418) -> ("error out"=w415:errorcluster, "DIO Ref Out"=w416:T5)  [unwired: 6 in]
        n150 = global write "Global_pH.vi" "Dangerous_Work"(TRUE ("Dangerous_Work")) -> ()
        n151 = global write "Global_pH.vi" "Work"(FALSE ("Dangerous_Work")) -> ()
        n152 = global write "Global_pH.vi" "FREE"(FALSE ("Dangerous_Work")) -> ()
      }
      frame "BACK" {
        n153 = Enqueue Element(queue=w432, element=state_R."Halt" ("State Selector"), error in (no error)=w431) -> ()  [unwired: 1 in, 3 out]
        n154 = call <vilib>:"Write.vi"("error in (no error)"=w428, "Values"=bool[] [TRUE, TRUE, FALSE, TRUE, TRUE, TRUE], "DIO Ref In"=w429) -> ("error out"=w426:errorcluster, "DIO Ref Out"=w427:T5)  [unwired: 6 in]
        n155 = global write "Global_pH.vi" "Dangerous_Work"(TRUE ("Dangerous_Work")) -> ()
        n156 = global write "Global_pH.vi" "Work"(FALSE ("Dangerous_Work")) -> ()
        n157 = global write "Global_pH.vi" "FREE"(FALSE ("Dangerous_Work")) -> ()
      }
      frame "Reset" {
        n158 = Enqueue Element(queue=w441, element=state_R."Initialize" ("State Selector"), error in (no error)=w440) -> ()  [unwired: 1 in, 3 out]
        n159 = call <vilib>:"Write.vi"("error in (no error)"=w436, "Values"=bool[] [TRUE, TRUE, TRUE, TRUE, TRUE, TRUE], "DIO Ref In"=w437) -> ("error out"=w434:errorcluster, "DIO Ref Out"=w435:T5)  [unwired: 6 in]
      }
      frame "Process" {
        n160 = Enqueue Element(queue=w446, element=state_R."Halt" ("State Selector"), error in (no error)=w445) -> ()  [unwired: 1 in, 3 out]
      }
      frame "PAUSE" {
        n161 = Enqueue Element(queue=w453, element=state_R."Halt" ("State Selector"), error in (no error)=w452) -> ()  [unwired: 1 in, 3 out]
        n162 = call <vilib>:"Write.vi"("error in (no error)"=w449, "Values"=bool[] [TRUE, TRUE, TRUE, TRUE, TRUE, TRUE], "DIO Ref In"=w450) -> ("error out"=w447:errorcluster, "DIO Ref Out"=w448:T5)  [unwired: 6 in]
      }
      frame "Report" {
        n163 = Enqueue Element(queue=w462, element=state_R."Halt" ("State Selector"), error in (no error)=w461) -> ()  [unwired: 1 in, 3 out]
        n164 = call <vilib>:"Write.vi"("error in (no error)"=w457, "Values"=bool[] [TRUE, TRUE, TRUE, TRUE, TRUE, TRUE], "DIO Ref In"=w458) -> ("error out"=w455:errorcluster, "DIO Ref Out"=w456:T5)  [unwired: 6 in]
      }
      frame "Halt" {
      }
      frame "Shutdown" {
        n165 = call <vilib>:"Write.vi"("error in (no error)"=w470, "Values"=bool[] [TRUE, TRUE, TRUE, TRUE, TRUE, TRUE], "DIO Ref In"=w471) -> ("error out"=w468:errorcluster, "DIO Ref Out"=w469:T5)  [unwired: 6 in]
        n166 = global write "Global_pH.vi" "Dangerous_Work"(FALSE ("Dangerous_Work")) -> ()
        n167 = global write "Global_pH.vi" "Work"(FALSE ("Dangerous_Work")) -> ()
        n168 = global write "Global_pH.vi" "FREE"(TRUE ("Dangerous_Work")) -> ()
      }
    }
    n169 = local read "程式終止"() -> (w257:bool)
    n170 = Wait (ms)(milliseconds to wait=u32 10) -> ()  [unwired: 1 out]
  }
  n171 = call <vilib>:"Close.vi"("error in (no error)"=w19, "DIO Ref In"=w20) -> ()  [unwired: 9 in, 1 out]
  n172 = call <vilib>:"daqio_Close.vi"("error in (no error)"=w2, "daq.io type"=w3) -> ()  [unwired: 9 in, 1 out]
  n173 = call <vilib>:"daqio_Close.vi"("error in (no error)"=w10, "daq.io type"=w11) -> ()  [unwired: 9 in, 1 out]
  n174 = call <vilib>:"daqio_Close.vi"("error in (no error)"=w8, "daq.io type"=w9) -> ()  [unwired: 9 in, 1 out]
  n175 = call <vilib>:"daqio_Close.vi"("error in (no error)"=w6, "daq.io type"=w7) -> ()  [unwired: 9 in, 1 out]
  n176 = call <vilib>:"Close.vi"("error in (no error)"=w23, "DIO Ref In"=w24) -> ()  [unwired: 9 in, 1 out]
  n177 = Release Queue(queue=w31, error in (no error)=w30) -> (error out=w29:errorcluster)  [unwired: 1 in, 2 out]
  n178 = call <vilib>:"Simple Error Handler.vi"("error in (no error)"=w29) -> ()  [unwired: 4 in, 5 out]
